vi "test1.vi"() -> ()   [LabVIEW 2013, in "std eng tests.lvlib"]
uses:
  std eng tests.lvlib
  <vilib>/NI/Module Execution Interface/Engine Runtime/Execution States.ctl
  Runtime/error responses.ctl
  Configuration/error options.ctl
  <vilib>/NI/Module Execution Interface/Engine Runtime/Fault.ctl
  <vilib>/NI/Tag Bus Module Framework/runtime/error classification.ctl
  Configuration/Standard Engine Configuration.lvclass
  Runtime/Standard Engine Runtime.lvclass
  <vilib>/NI/Tag Bus Module Framework/channel/channel classification.ctl
  Configuration/Module Decimation.ctl
  Configuration/Supported Timing Sources.ctl
  testmodule/execution/testmod runtime.lvclass
  testmodule/configuration/testmod configuration.lvclass
  <vilib>/NI/Tag Bus/tag/Data Type.ctl
  Configuration/timing reporting tags.ctl
  Configuration/Standard Engine Configuration.lvclass/Standard Engine Configuration.ctl
  testmodule/configuration/testmod configuration.lvclass/testmod configuration.ctl
  <vilib>/NI/Tag Bus/tag/tag descriptor.lvclass
  testmodule/configuration/Write channels.vi
  Configuration/Write Timing Source Type.vi
  Configuration/Write Timing Source dt.vi
  Configuration/Find Module Specific Config.vi
  <vilib>/NI/Configuration Framework/error generator.vi
  <vilib>/NI/Module Execution Interface/Engine Runtime/Engine Runtime Interface.lvclass
  <vilib>/NI/Tag Bus Module Framework/channel/TBM channel.lvclass
  <vilib>/NI/Module Execution Interface/Engine Configuration/engine configuration.lvclass
  <vilib>/NI/Configuration Framework/serializable configuration/NISE_CEF_serializable configuration.lvclass
  main engine/main engine.lvlib
  async executor/async executor.lvlib
  worker library/worker pool.lvlib
  <vilib>/NI/Tag Bus Module Framework/runtime/TBM module execution interface.lvclass
panel:
  in  "stop l2":bool
  out "faults":T1[](array[typedef])
  in  "error responses":T3={"unknown"={"clear"=FALSE, "notify"=TRUE, "remove module"=FALSE, "abort engine"=FALSE, "go to safe state"=TRUE, "recover module"=FALSE}, "trivial"={"clear"=FALSE, "notify"=TRUE, "remove module"=TRUE, "abort engine"=FALSE, "go to safe state"=FALSE, "recover module"=FALSE}, "critical"={"clear"=FALSE, "notify"=TRUE, "remove module"=FALSE, "abort engine"=TRUE, "go to safe state"=FALSE, "recover module"=FALSE}, "recoverable"={"clear"=FALSE, "notify"=TRUE, "remove module"=FALSE, "abort engine"=FALSE, "go to safe state"=FALSE, "recover module"=TRUE}}
  in  "async?":bool
  out "Engine State":T5
  in  "stop l3":bool
  out "final error":errorcluster
  in  "stop":bool
  out "runtime error":errorcluster
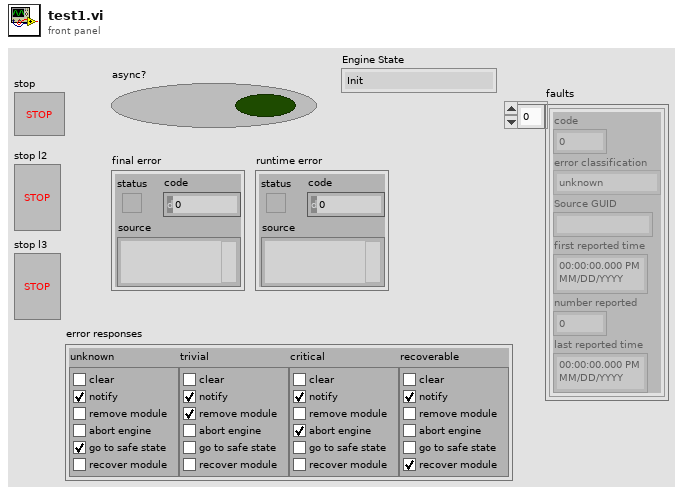
[diagram p1: front panel]
types:
  T1 = typedef "Engine Runtime Interface.lvclass/Fault.ctl" = cluster{"code":i32, "error classification":T2, "Source GUID":string, "first reported time":timestamp, "number reported":u32, "last reported time":timestamp}
  T2 = typedef "TBM module execution interface.lvclass/error classification.ctl" = enum16{"unknown", "none", "trivial", "recoverable", "critical"}
  T3 = typedef "Standard Engine Configuration.lvclass/error responses.ctl" = cluster{"unknown":T4, "trivial":T4, "critical":T4, "recoverable":T4}
  T4 = typedef "Standard Engine Configuration.lvclass/error options.ctl" = cluster{"clear":bool, "notify":bool, "remove module":bool, "abort engine":bool, "go to safe state":bool, "recover module":bool}
  T5 = typedef "Engine Runtime Interface.lvclass/Execution States.ctl" = enum16{"Init", "Pre-Operational", "Safe-Operational", "Operational", "Stopped"}
  T6 = typedef "tag bus.lvlib/tag descriptor.lvclass/Data Type.ctl" = enum16{"Double", "Single", "I64", "I32", "I16", "I8", "U64", "U32", "U16", "U8", "Boolean", "String", "Array of Double", "Array of Single", "Array of I64", "Array of I32", "Array of I16", "Array of I8", "Array of U64", "Array of U32", "Array of U16", "Array of U8", "Array of Boolean", "Array of String"}
  T7 = typedef "TBM channel.lvclass/channel classification.ctl" = enum16{"input data", "output data", "processing parameter", "processing result"}
  T8 = typedef "Standard Engine Configuration.lvclass/timing reporting tags.ctl" = cluster{"late index (bool)":string, "late count index (U32)":string, "current dt ns(U64)":string, "last exec time ns(U64)":string}
  T9 = typedef "Standard Engine Configuration.lvclass/Supported Timing Sources.ctl" = enum16{"Use Module Timing Source", "1 kHz Clock", "1 MHz Clock", "Synchronize to Scan Engine"}
  T10 = typedef "Standard Engine Configuration.lvclass/Module Decimation.ctl" = cluster{"Decimation":u16, "Offset":u16, "sort order":i32, "async?":bool}
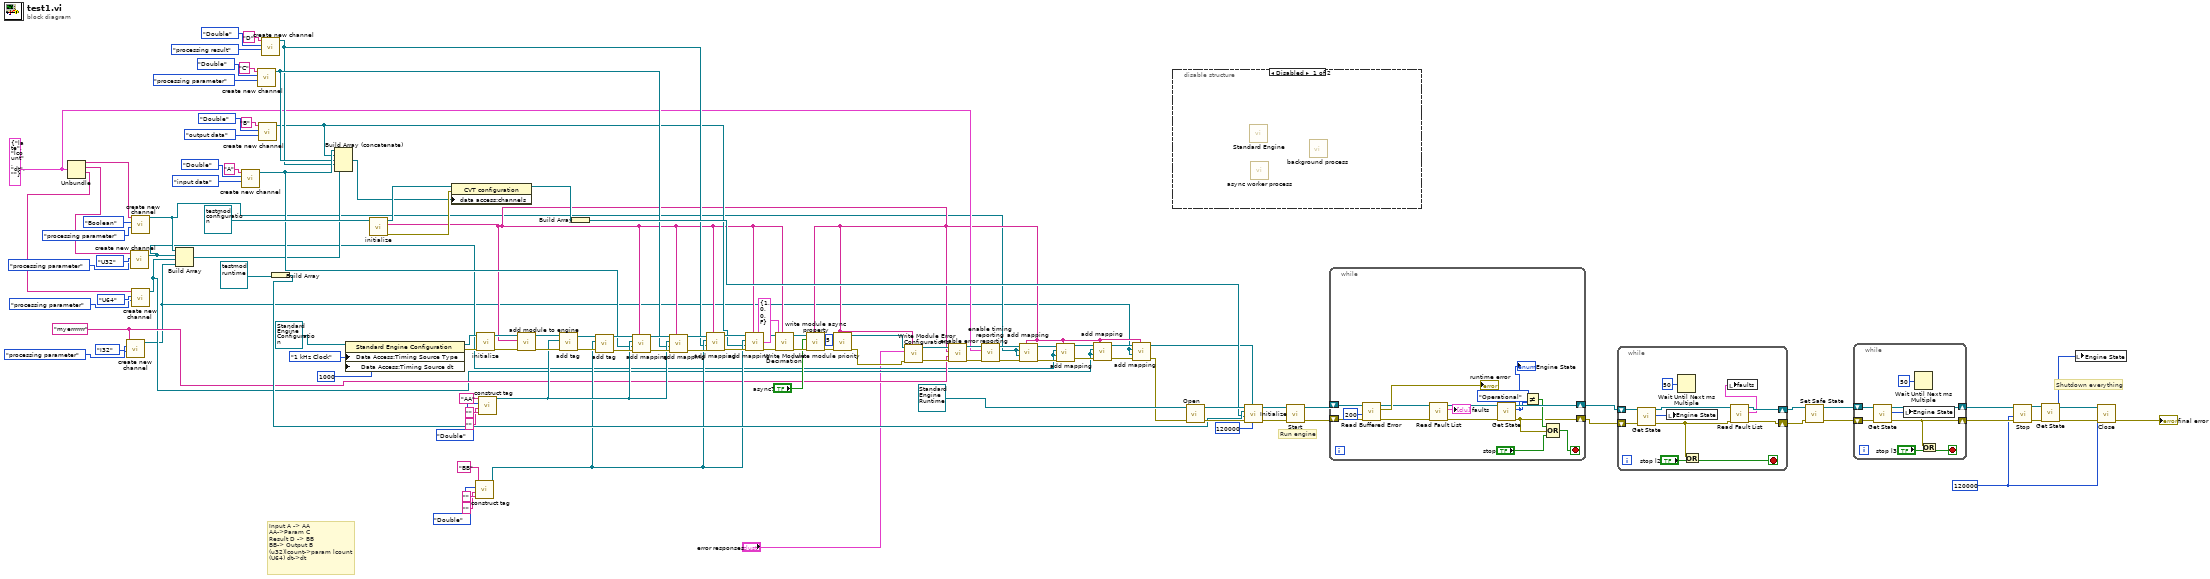
[diagram p0: block diagram]
diagram:
  w10 = 120000 ("timeout (-1)")
  w28 = "myerrrrrrr" ("channel name")
  w27 = T8 {"late index (bool)"="late", "late count index (U32)"="lcount", "current dt ns(U64)"="dt", "last exec time ns(U64)"=""} ("timing reporting")
  # "Input A -> AA\nAA->Param C\nResult D -> BB\nBB-> Output B\n(u32)lcount->param lcount\n(U64) dt->dt"
  # "Shutdown everything"
  # "Run engine"
  n1 = Unbundle(w27) -> ("late index (bool)"=w34:string, "late count index (U32)"=w33:string, "current dt ns(U64)"=w32:string)  [unwired: 1 out]
  n2 = call <vilib>:"create new channel.vi"("channel classification"=channel_classification."processing parameter", "data type"=Data_Type."I32", "channel name"=w28) -> ("channel"=w12:refnum<class "TBM channel.lvclass">)  [unwired: 8 in]
  n3 = call <vilib>:"create new channel.vi"("channel classification"=channel_classification."processing parameter", "data type"=Data_Type."U32", "channel name"=w33) -> ("channel"=w14:refnum<class "TBM channel.lvclass">)  [unwired: 8 in]
  n4 = call <vilib>:"create new channel.vi"("channel classification"=channel_classification."processing parameter", "data type"=Data_Type."Boolean", "channel name"=w34) -> ("channel"=w15:refnum<class "TBM channel.lvclass">)  [unwired: 8 in]
  n5 = call <vilib>:"create new channel.vi"("channel classification"=channel_classification."processing parameter", "data type"=Data_Type."U64", "channel name"=w32) -> ("channel"=w13:refnum<class "TBM channel.lvclass">)  [unwired: 8 in]
  n6 = Build Array(w15, w14, w13, w12) -> (w29:refnum<class "TBM channel.lvclass">[])
  n7 = call <vilib>:"create new channel.vi"("channel classification"=channel_classification."input data", "data type"=Data_Type."Double", "channel name"="A") -> ("channel"=w50:refnum<class "TBM channel.lvclass">)  [unwired: 8 in]
  n8 = call <vilib>:"create new channel.vi"("channel classification"=channel_classification."processing parameter", "data type"=Data_Type."Double", "channel name"="C") -> ("channel"=w49:refnum<class "TBM channel.lvclass">)  [unwired: 8 in]
  n9 = call <vilib>:"create new channel.vi"("channel classification"=channel_classification."output data", "data type"=Data_Type."Double", "channel name"="B") -> ("channel"=w47:refnum<class "TBM channel.lvclass">)  [unwired: 8 in]
  n10 = call <vilib>:"create new channel.vi"("channel classification"=channel_classification."processing result", "data type"=Data_Type."Double", "channel name"="D") -> ("channel"=w48:refnum<class "TBM channel.lvclass">)  [unwired: 8 in]
  n11 = Build Array(refnum<class "testmod runtime.lvclass"> refnum ("CVT runtime")) -> (w81:refnum<class "testmod runtime.lvclass">[])
  n12 = Build Array (concatenate)(w50, w47, w49, w48, w29) -> (w75:refnum<class "TBM channel.lvclass">[])
  n13 = property class="Standard Engine Configuration"(reference=refnum<class "Standard Engine Configuration.lvclass"> refnum ("Standard Engine Configuration"), "Data Access:Timing Source Type"=Supported_Timing_Sources."1 kHz Clock" ("Timing Source Type"), "Data Access:Timing Source dt"=u32 1000 ("Timing Source dt")) -> (reference out=w85:refnum<class "Standard Engine Configuration.lvclass">, error out=w87:errorcluster)  [unwired: 1 in]
  n14 = call <vilib>:"initialize.vi"("configuration in"=refnum<class "testmod configuration.lvclass"> refnum ("CVT configuration")) -> ("error out"=w78:errorcluster, "identifier"=w16:string, "configuration out"=w79:refnum<class "testmod configuration.lvclass">)  [unwired: 8 in]
  n15 = property class="CVT configuration"(reference=w79, error in=w78, "data access:channels"=w75) -> (reference out=w77:refnum<class "testmod configuration.lvclass">)  [unwired: 1 out]
  n16 = call <vilib>:"construct tag.vi"("raw default"="", "metadata"="", "data type"=Data_Type."Double", "name"="BB") -> ("system tag out"=w51:refnum<class "tag descriptor.lvclass">)  [unwired: 6 in, 1 out]
  n17 = call <vilib>:"initialize.vi"("error in"=w87, "configuration in"=w85) -> ("error out"=w103:errorcluster, "configuration out"=w102:refnum<class "Standard Engine Configuration.lvclass">)  [unwired: 7 in, 1 out]
  n18 = call <vilib>:"construct tag.vi"("raw default"="", "metadata"="", "data type"=Data_Type."Double", "name"="AA") -> ("system tag out"=w52:refnum<class "tag descriptor.lvclass">)  [unwired: 6 in, 1 out]
  n19 = call-dynamic "add module to engine.vi"("error in"=w103, "module ID"=w16, "Standard Engine Configuration in"=w102) -> ("error out"=w105:errorcluster, "Standard Engine Configuration out"=w104:refnum<class "Standard Engine Configuration.lvclass">)  [unwired: 7 in]
  n20 = call <vilib>:"add tag.vi"("error in"=w105, "tag descriptor"=w52, "engine configuration in"=w104) -> ("error out"=w67:errorcluster, "engine configuration out"=w68:refnum<class "Standard Engine Configuration.lvclass">)  [unwired: 7 in]
  n21 = Build Array(w77) -> (w76:refnum<class "testmod configuration.lvclass">[])
  n22 = call <vilib>:"add tag.vi"("error in"=w67, "tag descriptor"=w51, "engine configuration in"=w68) -> ("error out"=w66:errorcluster, "engine configuration out"=w54:refnum<class "Standard Engine Configuration.lvclass">)  [unwired: 7 in]
  n23 = call <vilib>:"add mapping.vi"("owner ID"=w16, "error in"=w66, "channel"=w50, "tag descriptor"=w52, "engine configuration"=w54) -> ("error out"=w55:errorcluster, "engine configuration out"=w53:refnum<class "Standard Engine Configuration.lvclass">)  [unwired: 5 in]
  n24 = call <vilib>:"add mapping.vi"("owner ID"=w16, "error in"=w55, "channel"=w49, "tag descriptor"=w52, "engine configuration"=w53) -> ("error out"=w57:errorcluster, "engine configuration out"=w56:refnum<class "Standard Engine Configuration.lvclass">)  [unwired: 5 in]
  n25 = call <vilib>:"add mapping.vi"("owner ID"=w16, "error in"=w57, "channel"=w48, "tag descriptor"=w51, "engine configuration"=w56) -> ("error out"=w107:errorcluster, "engine configuration out"=w106:refnum<class "Standard Engine Configuration.lvclass">)  [unwired: 5 in]
  n26 = call <vilib>:"add mapping.vi"("owner ID"=w16, "error in"=w107, "channel"=w47, "tag descriptor"=w51, "engine configuration"=w106) -> ("error out"=w98:errorcluster, "engine configuration out"=w99:refnum<class "Standard Engine Configuration.lvclass">)  [unwired: 5 in]
  n27 = call "Write Module Decimation.vi"("Module ID"=w16, "error in"=w98, "Module Decimation"=T10 {"Decimation"=1, "Offset"=0, "sort order"=0, "async?"=FALSE}, "Standard Engine Repo Data in"=w99) -> ("error out"=w100:errorcluster, "Standard Engine Repo Data out"=w101:refnum<class "Standard Engine Configuration.lvclass">)  [unwired: 6 in]
  n28 = call "write module async property.vi"("Module ID"=w16, "error in"=w100, "async?"="async?", "Standard Engine Repo Data in"=w101) -> ("error out"=w96:errorcluster, "Standard Engine Repo Data out"=w95:refnum<class "Standard Engine Configuration.lvclass">)  [unwired: 6 in]
  n29 = call "write module priority.vi"("Module ID"=w16, "error in"=w96, "execution order priority"=5, "Standard Engine Repo Data in"=w95) -> ("error out"=w41:errorcluster, "Standard Engine Repo Data out"=w46:refnum<class "Standard Engine Configuration.lvclass">)  [unwired: 6 in]
  n30 = call "Write Module Error Configurations.vi"("Module ID"=w16, "error in"=w41, "error responses"="error responses", "Standard Engine Repo Data in"=w46) -> ("error out"=w42:errorcluster, "Standard Engine Repo Data out"=w45:refnum<class "Standard Engine Configuration.lvclass">)  [unwired: 6 in]
  n31 = call "enable error reporting.vi"("error in"=w42, "tag"=w28, "module ID"=w16, "Standard Engine Configuration in"=w45) -> ("error out"=w43:errorcluster, "Standard Engine Configuration out"=w44:refnum<class "Standard Engine Configuration.lvclass">)  [unwired: 6 in]
  n32 = call "enable timing reporting.vi"("error in"=w43, "timing reporting"=w27, "Standard Engine Configuration in"=w44) -> ("error out"=w19:errorcluster, "Standard Engine Configuration out"=w20:refnum<class "Standard Engine Configuration.lvclass">)  [unwired: 7 in]
  n33 = call <vilib>:"add mapping.vi"("owner ID"=w16, "error in"=w19, "channel"=w15, "tag descriptor"=w15, "engine configuration"=w20) -> ("error out"=w25:errorcluster, "engine configuration out"=w26:refnum<class "Standard Engine Configuration.lvclass">)  [unwired: 5 in]
  n34 = call <vilib>:"add mapping.vi"("owner ID"=w16, "error in"=w25, "channel"=w14, "tag descriptor"=w14, "engine configuration"=w26) -> ("error out"=w23:errorcluster, "engine configuration out"=w24:refnum<class "Standard Engine Configuration.lvclass">)  [unwired: 5 in]
  n35 = call <vilib>:"add mapping.vi"("owner ID"=w16, "error in"=w23, "channel"=w13, "tag descriptor"=w13, "engine configuration"=w24) -> ("error out"=w21:errorcluster, "engine configuration out"=w22:refnum<class "Standard Engine Configuration.lvclass">)  [unwired: 5 in]
  n36 = call <vilib>:"add mapping.vi"("owner ID"=w16, "error in"=w21, "channel"=w12, "tag descriptor"=w12, "engine configuration"=w22) -> ("error out"=w18:errorcluster, "engine configuration out"=w17:refnum<class "Standard Engine Configuration.lvclass">)  [unwired: 5 in]
  n37 = disable-structure shown="Disabled" {
    frame Disabled {
      n38 = call "Standard Engine.vi"() -> ()  [unwired: 12 in]
      n39 = call "async worker process.vi"() -> ()  [unwired: 9 in, 3 out]
      n40 = call "background process.vi"() -> ()  [unwired: 12 in]
    }
    frame Enabled {
    }
  }
  n41 = call-dynamic "Open.vi"("error in"=w18, "Standard Engine Runtime in"=refnum<class "Standard Engine Runtime.lvclass"> refnum ("Standard Engine Runtime")) -> ("error out"=w117:errorcluster, "Standard Engine Runtime out"=w118:refnum<class "Standard Engine Runtime.lvclass">)  [unwired: 8 in]
  n42 = call-dynamic <vilib>:"Initialize.vi"("timeout in ms"=120000, "Engine Configuration"=w17, "error in"=w117, "Module Configurations"=w76, "Modules"=w81, "Standard Engine Runtime in"=w118) -> ("error out"=w116:errorcluster, "Standard Engine Runtime out"=w115:refnum<class "Standard Engine Runtime.lvclass">)  [unwired: 4 in]
  n43 = call-dynamic "Start.vi"("error in"=w116, "Standard Engine Runtime in"=w115) -> ("error out"=w120:errorcluster, "Standard Engine Runtime out"=w121:refnum<class "Standard Engine Runtime.lvclass">)  [unwired: 8 in]
  n44 = while {
    shift-right: [w134] -> w1
    shift-left: w121 -> [w137]
    shift-right: [w128] -> w2
    shift-left: w120 -> [w136]
    stop <- w132 stop-if-true
    n45 = call-dynamic "Read Buffered Error.vi"("error in"=w136, "timeout in ms (0)"=200, "Standard Engine Runtime in"=w137) -> ("error out"=w135:errorcluster, "Engine Error"=→"runtime error":errorcluster, "Standard Engine Runtime out"=w124:refnum<class "Standard Engine Runtime.lvclass">)  [unwired: 6 in]
    n46 = call-dynamic "Read Fault List.vi"("error in"=w135, "Standard Engine Runtime in"=w124) -> ("error out"=w125:errorcluster, "faults"=→"faults":T1[], "Standard Engine Runtime out"=w123:refnum<class "Standard Engine Runtime.lvclass">)  [unwired: 7 in]
    n47 = call-dynamic "Get State.vi"("error in"=w125, "Standard Engine Runtime in"=w123) -> ("error out"=w128:errorcluster, "Engine State"=w126:T5, "Standard Engine Runtime out"=w134:refnum<class "Standard Engine Runtime.lvclass">)  [unwired: 7 in]
    "Engine State" <- w126
    n48 = Not Equal?(x=Execution_States."Operational" ("Engine State"), y=w126) -> (x != y?=w129:bool)
    n49 = Compound Arithmetic op=OR(w129, w128, "stop") -> (w132:bool)
  }
  n50 = while {
    shift-right: [w139] -> w4
    shift-left: w1 -> [w147]
    shift-right: [w140] -> w3
    shift-left: w2 -> [w148]
    stop <- w144 stop-if-true
    n51 = call-dynamic "Get State.vi"("error in"=w148, "Standard Engine Runtime in"=w147) -> ("error out"=w141:errorcluster, "Engine State"=w143:T5, "Standard Engine Runtime out"=w142:refnum<class "Standard Engine Runtime.lvclass">)  [unwired: 7 in]
    n52 = local write "Engine State"(w143) -> ()
    n53 = Wait Until Next ms Multiple(millisecond multiple=u32 50) -> ()  [unwired: 1 out]
    n54 = Or(x=w141, y="stop l2") -> (x .or. y?=w144:bool)
    n55 = call-dynamic "Read Fault List.vi"("error in"=w141, "Standard Engine Runtime in"=w142) -> ("error out"=w140:errorcluster, "faults"=w138:T1[], "Standard Engine Runtime out"=w139:refnum<class "Standard Engine Runtime.lvclass">)  [unwired: 7 in]
    n56 = local write "faults"(w138) -> ()
  }
  n57 = call-dynamic "Set Safe State.vi"("error in"=w3, "Standard Engine Runtime in"=w4) -> ("error out"=w89:errorcluster, "Standard Engine Runtime out"=w88:refnum<class "Standard Engine Runtime.lvclass">)  [unwired: 8 in]
  n58 = while {
    shift-right: [w154] -> w90
    shift-left: w88 -> [w155]
    shift-right: [w150] -> w91
    shift-left: w89 -> [w156]
    stop <- w151 stop-if-true
    n59 = call-dynamic "Get State.vi"("error in"=w156, "Standard Engine Runtime in"=w155) -> ("error out"=w150:errorcluster, "Engine State"=w149:T5, "Standard Engine Runtime out"=w154:refnum<class "Standard Engine Runtime.lvclass">)  [unwired: 7 in]
    n60 = local write "Engine State"(w149) -> ()
    n61 = Wait Until Next ms Multiple(millisecond multiple=u32 50) -> ()  [unwired: 1 out]
    n62 = Or(x=w150, y="stop l3") -> (x .or. y?=w151:bool)
  }
  n63 = call-dynamic "Stop.vi"("error in"=w91, "timeout (-1)"=w10, "Standard Engine Runtime in"=w90) -> ("error out"=w7:errorcluster, "Standard Engine Runtime out"=w8:refnum<class "Standard Engine Runtime.lvclass">)  [unwired: 7 in]
  n64 = call-dynamic "Get State.vi"("error in"=w7, "Standard Engine Runtime in"=w8) -> ("error out"=w6:errorcluster, "Engine State"=w9:T5, "Standard Engine Runtime out"=w5:refnum<class "Standard Engine Runtime.lvclass">)  [unwired: 7 in]
  n65 = local write "Engine State"(w9) -> ()
  n66 = call-dynamic "Close.vi"("error in"=w6, "timeout (-1)"=w10, "Standard Engine Runtime in"=w5) -> ("error out"=→"final error":errorcluster)  [unwired: 8 in]
